vi "tol to color converter.vi"(2 "Tolerancia":T1) -> (6 "Color":u32(colorbox))   [LabVIEW 2018]
uses:
  Banda Tolerancia--control.ctl
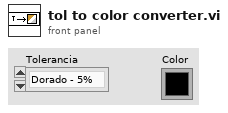
[diagram p1: front panel]
types:
  T1 = typedef "Banda Tolerancia--control.ctl" = enum16{"Dorado - 5%", "Plata - 10%"}
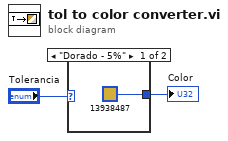
[diagram p0: block diagram]
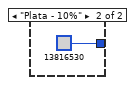
[diagram p2: hidden frame]
diagram:
  n1 = case shown="\"Dorado - 5%\"" "Tolerancia" {
    tunnel: [u32 13938487 u32 13816530] -> w1
    frame "Dorado - 5%" {
    }
    frame "Plata - 10%" {
    }
  }
  "Color" <- w1
